vi "Computer Play One Step.vi"(7 "board":u16[][](array[numeric]), 11 "Available White Position":i32[][](array[numeric])) -> (1 "column":i32, 2 "row":i32)   [LabVIEW 2018]
doc: "本VI是为《我和LabVIEW》一书编写的示例。\n关于本书的介绍请参考网页：\nhttp://ruanqizhen.spaces.live.com/blog/cns!5852D4F797C53FB6!4310.entry"
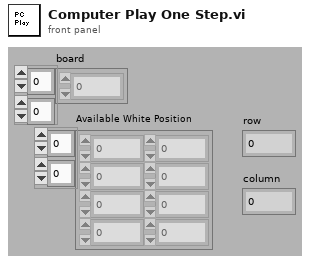
[diagram p1: front panel]
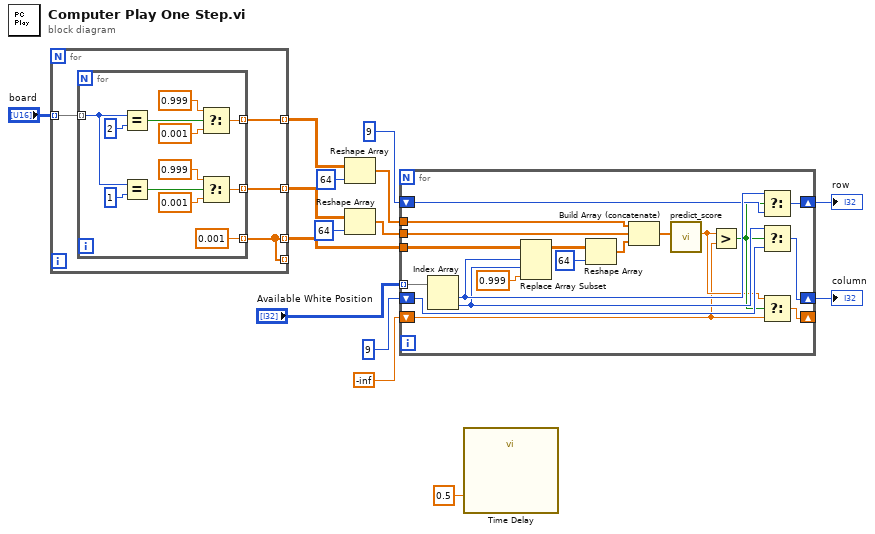
[diagram p0: block diagram]
diagram:
  n1 = for {
    tunnel: "board" -> [w19] mode=indexing
    tunnel: [w18] -> w13 mode=indexing
    tunnel: [w17] -> w11 mode=indexing
    tunnel: [w16] -> _ mode=indexing
    tunnel: [w16] -> w9 mode=indexing
    n2 = for {
      tunnel: w19 -> [w22] mode=indexing
      tunnel: [w27] -> w18 mode=indexing
      tunnel: [w21] -> w17 mode=indexing
      tunnel: [0.001 ("t")] -> w16 mode=indexing
      n3 = Equal?(x=w22, y=u16 2) -> (x = y?=w30:bool)
      n4 = Equal?(x=w22, y=u16 1) -> (x = y?=w24:bool)
      n5 = Select(t=0.999, s=w30, f=0.001 ("t")) -> (s? t:f=w27:dbl)
      n6 = Select(t=0.999, s=w24, f=0.001 ("t")) -> (s? t:f=w21:dbl)
    }
  }
  n7 = Reshape Array(w13, 64 ("dimension size")) -> (w12:dbl[])
  n8 = Reshape Array(w11, 64 ("dimension size")) -> (w10:dbl[])
  n9 = for {
    tunnel: "Available White Position" -> [w49] mode=indexing
    tunnel: w12 -> [w46]
    tunnel: w10 -> [w45]
    tunnel: w9 -> [w50]
    shift-right: [w33] -> _
    shift-left: -inf -> [w34]
    shift-right: [w41] -> w5
    shift-left: 9 ("row") -> [w38]
    shift-right: [w39] -> w4
    shift-left: 9 ("column") -> [w37]
    n10 = Index Array(array=w49) -> (element #1=w42:i32, element #2=w40:i32)  [unwired: 2 in]
    n11 = Replace Array Subset(array=w50, new element=0.999 ("t"), index (row)=w42, index (col)=w40) -> (w47:dbl[][])
    n12 = Reshape Array(w47, 64 ("dimension size")) -> (w44:dbl[])
    n13 = Build Array (concatenate)(w46, w45, w44) -> (w43:dbl[])
    n14 = call "predict_score.vi"("feature"=w43) -> ("predict"=w35:dbl)  [unwired: 10 in]
    n15 = Greater?(x=w35, y=w34) -> (0:w36:bool)
    n16 = Select(t=w42, s=w36, f=w38) -> (s? t:f=w41:i32)
    n17 = Select(t=w40, s=w36, f=w37) -> (s? t:f=w39:i32)
    n18 = Select(t=w35, s=w36, f=w34) -> (s? t:f=w33:dbl)
  }
  "column" <- w4
  "row" <- w5
  n19 = call "Time Delay"("Delay Time (s)"=0.5) -> ()  [unwired: 10 in, 1 out]
